vi "process_main.vi"(7 "FGV_mods":enum16{"Init", "Exec", "End"}(ring)=enum."Exec", 8 "Error In":errorcluster, 11 "DataIn":variant) -> (0 "Error Out":errorcluster)   [LabVIEW 2016]
uses:
  process_data.ctl
  MainFGV/Settings/Advanced/AdvancedConfig.ctl
  MainFGV/MainFGV_data.ctl
  MainFGV/Settings/config_board.ctl
  processing_mods.ctl
  Log/log_mods.ctl
  <vilib>/Analysis/5stat.llb/RMS (DBL).vi
  <vilib>/Analysis/NI_AALPro.lvlib
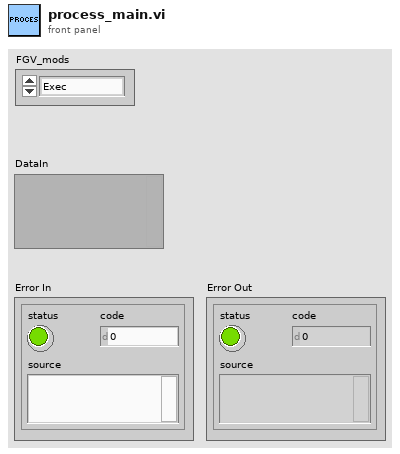
[diagram p1: front panel]
types:
  T1 = typedef "processing_mods.ctl" = enum16{"newData", "SetConfig", "setHammer"}
  T2 = typedef "MainFGV_data.ctl" = cluster{"TestDir":path, "TestName":string, "task":refnum<k21>, "data_file":refnum<file>, "AcqQueue":refnum<queue>, "StartTime":timestamp, "config_channels":T3[], "DAQmx Device":tag, "Advanced":T4, "running":bool, "hammerIndex":i32}
  T3 = typedef "config_board.ctl" = cluster{"Sens 1":dbl, "active 1":bool, "type 1":bool, "type 2":bool, "active 2":bool, "Sens 2":dbl, "type 3":bool, "active 3":bool, "Sens 3":dbl, "type 4":bool, "active 4":bool, "Sens 4":dbl}
  T4 = typedef "AdvancedConfig.ctl" = cluster{"rate":dbl, "duration":dbl, "thr":dbl, "preTrigger":dbl, "cutoff":dbl, "Filtro":enum16{"Desativado", "Passa banda", "Passa alta", "Passa baixa"}, "highPass":dbl, "lowPass":dbl, "updateTime":dbl}
  T5 = typedef "process_data.ctl" = cluster{"AcqQueue":refnum<queue>, "Advanced":T4, "refHammer":refnum<vi>, "refAcel":refnum<vi>, "hammerIndex":i32}
  T6 = typedef "log_mods.ctl" = enum16{"Init", "SetStatus", "RMSacel", "HitData", "Clear", "PeakForce", "WriteToLog", "End"}
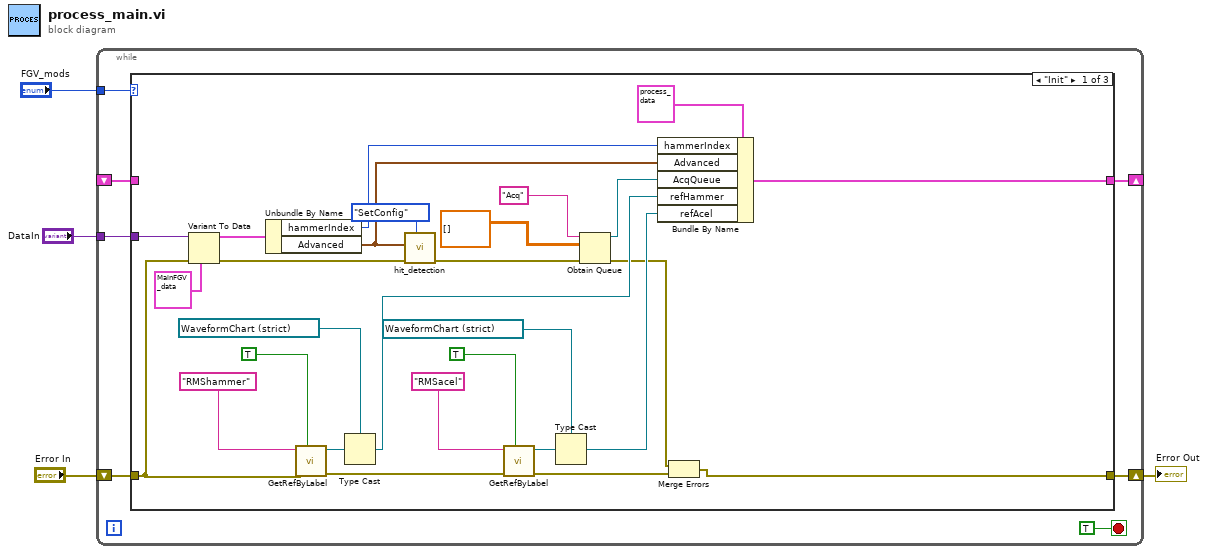
[diagram p0: block diagram]
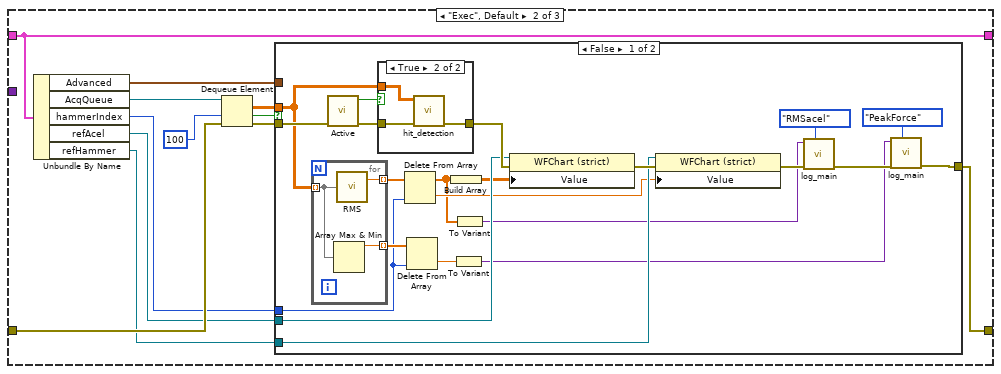
[diagram p2: hidden frame]
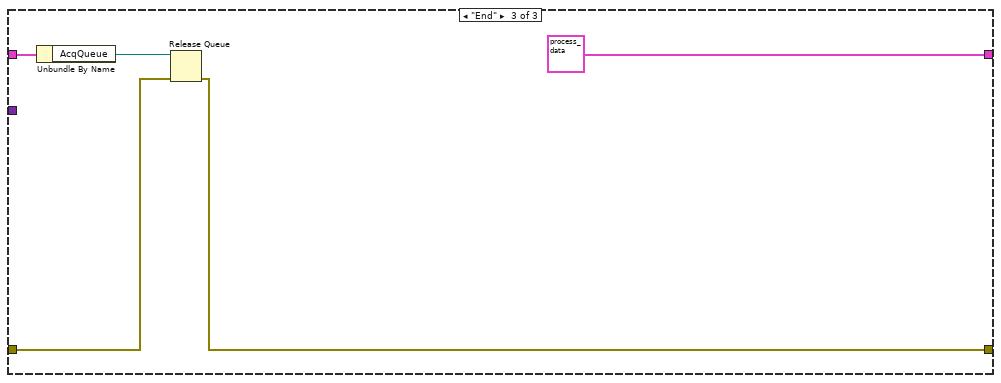
[diagram p5: hidden frame]
diagram:
  n1 = while {
    tunnel: "DataIn" -> [w10]
    tunnel: "FGV_mods" -> [w9]
    shift-right: [w8] -> _
    shift-left: _ -> [w7]
    shift-right: [w5] -> w1
    shift-left: "Error In" -> [w6]
    stop <- TRUE stop-if-true
    n2 = case shown="\"Init\"" w9 {
      tunnel: w10 -> [w39 _ _]
      tunnel: [w36 w51 T5 {"AcqQueue"=refnum, "Advanced"={"rate"=0.0, "duration"=1.0, "thr"=100.0, "preTrigger"=100.0, "cutoff"=-3.0, "Filtro"=enum."Desativado", "highPass"=1000.0, "lowPass"=1000.0, "updateTime"=50.0}, "refHammer"=refnum, "refAcel"=refnum, "hammerIndex"=0} ("process_data")] -> w8
      tunnel: w7 -> [_ w51 w86]
      tunnel: w6 -> [w20 w48 w83]
      tunnel: [w13 w44 w82] -> w5
      frame "Init" {
        n3 = Variant To Data(error in=w20, type=T2 {"TestDir"=path "", "TestName"="", "task"="", "data_file"=refnum, "AcqQueue"=refnum, "StartTime"=timestamp(0 s since 1904-01-01), "config_channels"=[], "DAQmx Device"="", "Advanced"={"rate"=1652.0, "duration"=1.0, "thr"=100.0, "preTrigger"=100.0, "cutoff"=-3.0, "Filtro"=enum."Desativado", "highPass"=1000.0, "lowPass"=1000.0, "updateTime"=50.0}, "running"=FALSE, "hammerIndex"=0} ("MainFGV_data"), Variant=w39) -> (data=w32:T2, error out=w30:errorcluster)
        n4 = Unbundle By Name(w32) -> ("hammerIndex"=w12:i32, "Advanced"=w31:T4)
        n5 = call "GetRefByLabel.vi"("InsideTab"=TRUE, "error in"=w20, "Label"="RMShammer") -> ("error out"=w22:errorcluster, "Ctl Refnum"=w25:refnum<vi>)  [unwired: 6 in, 1 out]
        n6 = Type Cast(type=refnum<vi> refnum ("RMShammer"), x=w25) -> (*(type *) &x=w16:refnum<vi>)
        n7 = call "hit_detection.vi"("mod"=processing_mods."SetConfig", "error in"=w30, "config"=w31) -> ("error out"=w29:errorcluster)  [unwired: 8 in]
        n8 = call "GetRefByLabel.vi"("InsideTab"=TRUE, "error in"=w22, "Label"="RMSacel") -> ("error out"=w15:errorcluster, "Ctl Refnum"=w21:refnum<vi>)  [unwired: 6 in, 1 out]
        n9 = Type Cast(type=refnum<vi> refnum ("RMSacel"), x=w21) -> (*(type *) &x=w17:refnum<vi>)
        n10 = Obtain Queue(name (unnamed)="Acq", element data type=dbl[][] [] ("2D array"), error in (no error)=w29) -> (queue out=w33:refnum<queue>, error out=w14:errorcluster)  [unwired: 2 in, 1 out]
        n11 = Bundle By Name(cluster=T5 {"AcqQueue"=refnum, "Advanced"={"rate"=0.0, "duration"=1.0, "thr"=100.0, "preTrigger"=100.0, "cutoff"=-3.0, "Filtro"=enum."Desativado", "highPass"=1000.0, "lowPass"=1000.0, "updateTime"=50.0}, "refHammer"=refnum, "refAcel"=refnum, "hammerIndex"=0} ("process_data"), "hammerIndex"=w12, "Advanced"=w31, "AcqQueue"=w33, "refHammer"=w16, "refAcel"=w17) -> (w36:T5)
        n12 = Merge Errors(w14, w15) -> (w13:errorcluster)
      }
      frame "Exec", Default {
        n13 = Unbundle By Name(w51) -> ("Advanced"=w43:T4, "AcqQueue"=w50:refnum<queue>, "hammerIndex"=w42:i32, "refAcel"=w41:refnum<vi>, "refHammer"=w40:refnum<vi>)
        n14 = Dequeue Element(queue=w50, timeout in ms (-1)=100, error in (no error)=w48) -> (element=w49:dbl[][], timed out?=w46:bool, error out=w45:errorcluster)  [unwired: 1 out]
        n15 = case shown="False" w46 {
          tunnel: w49 -> [w70 _]
          tunnel: w45 -> [w73 w81]
          tunnel: [w52 w81] -> w44
          tunnel: w43 -> [_ _]
          tunnel: w42 -> [w61 _]
          tunnel: w41 -> [w67 _]
          tunnel: w40 -> [w64 _]
          frame False {
            n16 = for {
              tunnel: w70 -> [w75] mode=indexing
              tunnel: [w76] -> w69 mode=indexing
              tunnel: [w74] -> w62 mode=indexing
              n17 = Array Max & Min(array=w75) -> (max value=w74:dbl)  [unwired: 3 out]
              n18 = call-poly <vilib>:"RMS.vi"("X"=w75) -> ("rms value"=w76:dbl)  [unwired: 1 out]
            }
            n19 = call "Active.vi"("Error In"=w73) -> ("Error Out"=w72:errorcluster, "active"=w71:bool)  [unwired: 9 in]
            n20 = case shown="True" w71 {
              tunnel: w70 -> [_ w80]
              tunnel: [w77 w79] -> w68
              tunnel: w72 -> [w77 w78]
              frame False {
              }
              frame True {
                n21 = call "hit_detection.vi"("error in"=w78, "data"=w80) -> ("error out"=w79:errorcluster)  [unwired: 9 in]
              }
            }
            n22 = Delete From Array(array=w69, index=w61) -> (deleted portion=w63:dbl, array with subset deleted=w58:dbl[])  [unwired: 1 in]
            n23 = Delete From Array(array=w62, index=w61) -> (deleted portion=w54:dbl)  [unwired: 1 in, 1 out]
            n24 = Build Array(w58) -> (w66:dbl[][])
            n25 = To Variant(anything=w54) -> (Variant=w53:variant)
            n26 = To Variant(anything=w58) -> (Variant=w57:variant)
            n27 = property class="WFChart (strict)"(reference=w67, error in=w68, "Value"=w66) -> (error out=w65:errorcluster)  [unwired: 1 out]
            n28 = property class="WFChart (strict)"(reference=w64, error in=w65, "Value"=w63) -> (error out=w59:errorcluster)  [unwired: 1 out]
            n29 = call "log_main.vi"("FGV_mods"=log_mods."RMSacel", "Error In"=w59, "DataIn"=w57) -> ("Error Out"=w55:errorcluster)  [unwired: 8 in]
            n30 = call "log_main.vi"("FGV_mods"=log_mods."PeakForce", "Error In"=w55, "DataIn"=w53) -> ("Error Out"=w52:errorcluster)  [unwired: 8 in]
          }
          frame True {
          }
        }
      }
      frame "End" {
        n31 = Unbundle By Name(w86) -> ("AcqQueue"=w85:refnum<queue>)
        n32 = Release Queue(queue=w85, error in (no error)=w83) -> (error out=w82:errorcluster)  [unwired: 1 in, 2 out]
      }
    }
  }
  "Error Out" <- w1
